vi "Scan Setup.vi"(8 "error in (no error)":errorcluster, 11 "Instrument in":refnum<class "Instrument.lvclass">) -> (0 "error out":errorcluster, 1 "User Cancelled?":bool, 3 "Instrument out":refnum<class "Instrument.lvclass">)   [LabVIEW 2009, in "Instrument.lvclass"]
doc: "(Dynamic) Send commands to configure the instrument according to the class member fields."
uses:
  Instrument.lvclass
  LCD/LCD Retarder.lvclass
  Scanners/Analog Out Scan/Analog Out Scan.lvclass
  Scanners/Function Gen Scan/Function Gen Scan.lvclass
  Scanners/Pulse Gen Basic Scan/Pulse Gen Basic Scan.lvclass
  Scanners/Pulse Gen Scan/Pulse Gen Scan.lvclass
  Scanners/Scanner/Scanner.lvclass
  Scanners/Translation Stage/Translation Stage.lvclass
  Scanners/Wavelength/Wavelength.lvclass
  Scanners/Wavelength Digikröm/Wavelength Digikröm.lvclass
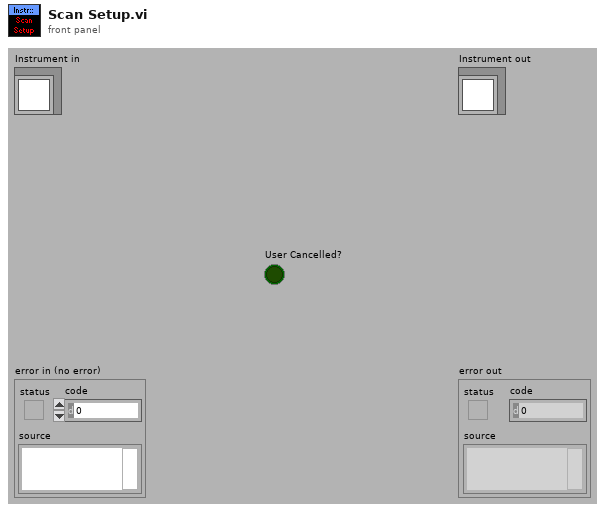
[diagram p1: front panel]
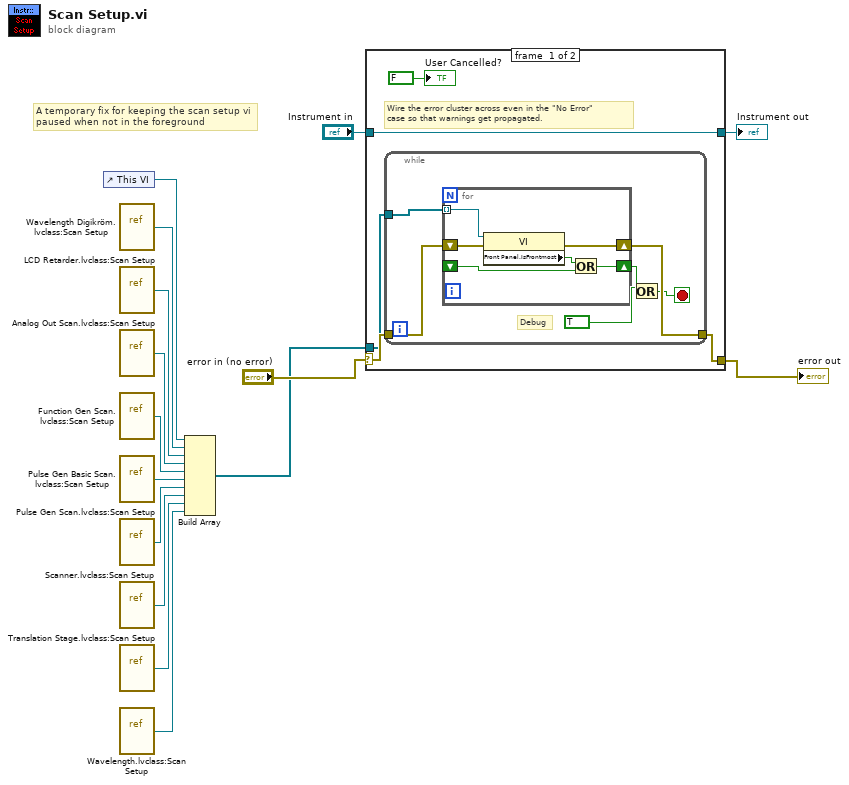
[diagram p0: block diagram]
diagram:
  # "A temporary fix for keeping the scan setup vi \npaused when not in the foreground"
  n1 = control-ref of="This VI"() -> (w1:refnum<vi>)
  n2 = vi-ref "Wavelength Digikröm.lvclass:Scan Setup.vi"() -> (w3:refnum<vi>)
  n3 = vi-ref "LCD Retarder.lvclass:Scan Setup.vi"() -> (w2:refnum<vi>)
  n4 = vi-ref "Analog Out Scan.lvclass:Scan Setup.vi"() -> (w10:refnum<vi>)
  n5 = vi-ref "Function Gen Scan.lvclass:Scan Setup.vi"() -> (w9:refnum<vi>)
  n6 = vi-ref "Pulse Gen Basic Scan.lvclass:Scan Setup.vi"() -> (w8:refnum<vi>)
  n7 = vi-ref "Pulse Gen Scan.lvclass:Scan Setup.vi"() -> (w7:refnum<vi>)
  n8 = vi-ref "Scanner.lvclass:Scan Setup.vi"() -> (w6:refnum<vi>)
  n9 = vi-ref "Translation Stage.lvclass:Scan Setup.vi"() -> (w5:refnum<vi>)
  n10 = vi-ref "Wavelength.lvclass:Scan Setup.vi"() -> (w4:refnum<vi>)
  n11 = Build Array(w1, w3, w2, w10, w9, w8, w7, w6, w5, w4) -> (w11:refnum<vi>[])
  n12 = case shown="No Error" "error in (no error)" {
    selector: "error in (no error)" -> [w18 w34]
    tunnel: [w17 w34] -> w14
    tunnel: [w19 w33] -> w12
    tunnel: "Instrument in" -> [w19 w33]
    tunnel: w11 -> [w16 _]
    frame #0 {
      # "Wire the error cluster across even in the \"No Error\"\ncase so that warnings get propagated."
      n13 = while {
        tunnel: [w26] -> w17
        tunnel: w16 -> [w25]
        tunnel: w18 -> [w24]
        stop <- w22 stop-if-true
        # "Debug"
        n14 = for {
          tunnel: w25 -> [w31] mode=indexing
          shift-right: [w32] -> w26
          shift-left: w24 -> [w30]
          shift-right: [w28] -> w23
          shift-left: _ -> [w27]
          n15 = property class="VI"(reference=w31, error in=w30) -> (error out=w32:errorcluster, "Front Panel.IsFrontmost"=w29:bool)  [unwired: 1 out]
          n16 = Or(x=w29, y=w27) -> (x .or. y?=w28:bool)
        }
        n17 = Or(x=TRUE, y=w23) -> (x .or. y?=w22:bool)
      }
      "User Cancelled?" <- FALSE ("User Cancelled?")
    }
    frame #1 {
    }
  }
  "error out" <- w14
  "Instrument out" <- w12
